vi "Save Data to TDMS File.vi"(8 "error in (no error)":errorcluster caption="错误输入（无错误）", 11 "Waveform Data Array":waveform(sgl)[](array[waveform]) caption="波形数组") -> (0 "error out":errorcluster caption="错误输出", 1 "Completed file path":path caption="完成文件路径")   [LabVIEW 2015]
doc: "读取DMA FIFO的波形数据。"
uses:
  <vilib>/Waveform/WDTOps.llb/WDT Index Channel DBL.vi
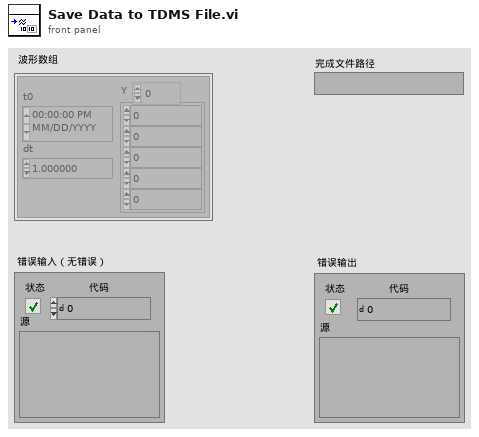
[diagram p1: front panel]
types:
  T1 = enum16{"Create New File", "Write File", "Close File"}
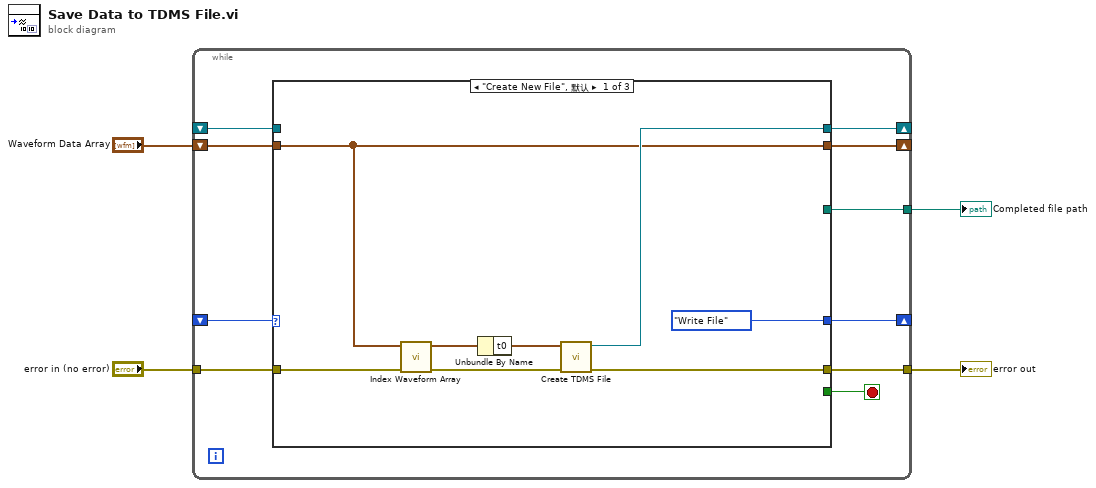
[diagram p0: block diagram]
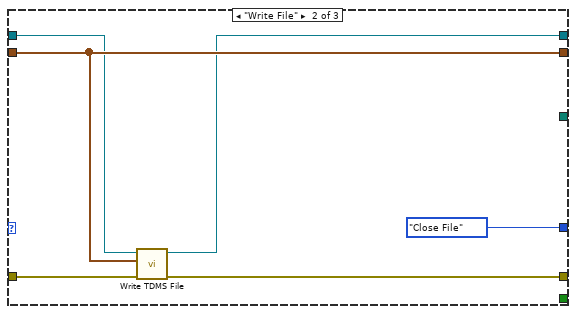
[diagram p2: hidden frame]
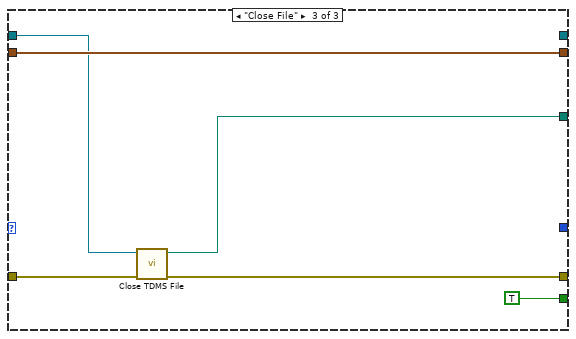
[diagram p3: hidden frame]
diagram:
  n1 = while {
    tunnel: "error in (no error)" -> [w13]
    tunnel: [w10] -> w2
    shift-right: [w11] -> _
    shift-left: _ -> [w12]
    shift-right: [w9] -> _
    shift-left: "Waveform Data Array" -> [w14]
    shift-right: [w7] -> _
    shift-left: _ -> [w8]
    tunnel: [w5] -> w1
    stop <- w6 stop-if-true
    n2 = case shown="\"Create New File\", 默认" w8 {
      tunnel: w14 -> [w18 w25 w32]
      tunnel: w13 -> [w17 w26 w34]
      tunnel: w12 -> [_ w24 w30]
      tunnel: [w21 w23 _] -> w11
      tunnel: [w20 w27 w33] -> w10
      tunnel: [w18 w25 w32] -> w9
      tunnel: [_ _ w31] -> w5
      tunnel: [T1."Write File" T1."Close File" _] -> w7
      tunnel: [_ _ TRUE] -> w6
      frame "Create New File", Default {
        n3 = call-poly <vilib>:"Index Waveform Array.vi"("error in (no error)"=w17, "waveform array"=w18) -> ("error out"=w16:errorcluster, "waveform"=w15:waveform(dbl))  [unwired: 8 in]
        n4 = Unbundle By Name(w15) -> ("t0"=w22:timestamp)
        n5 = call "Create TDMS File.vi"("error in (no error)"=w16, "Timestamp"=w22) -> ("error out"=w20:errorcluster, "TDMS File Reference"=w21:refnum<k34>)  [unwired: 8 in]
      }
      frame "Write File" {
        n6 = call "Write TDMS File.vi"("error in (no error)"=w26, "waveform array"=w25, "tdms file ref in"=w24) -> ("error out"=w27:errorcluster, "tdms file ref out"=w23:refnum<k34>)  [unwired: 7 in]
      }
      frame "Close File" {
        n7 = call "Close TDMS File.vi"("error in (no error)"=w34, "Log File"=w30) -> ("error out"=w33:errorcluster, "file path"=w31:path)  [unwired: 8 in]
      }
    }
  }
  "error out" <- w2
  "Completed file path" <- w1
